vi "Estrai DB DW Contigui.vi"(10 "DB REAL LETTURE":T1(array[cluster])) -> (1 "DBW number":i32[](array[numeric]), 2 "DB offset":i32[](array[numeric]), 3 "DB":i16[](array[numeric]))   [LabVIEW 2019]
panel:
  out "x = y?":bool
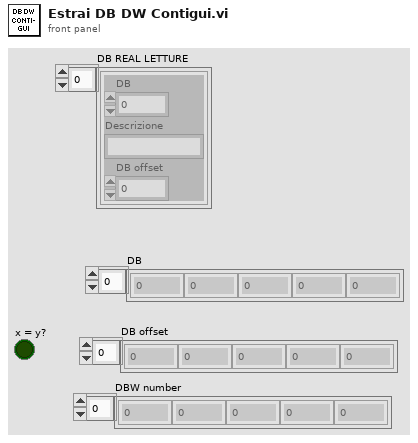
[diagram p1: front panel]
types:
  T1 = cluster{"DB":i16, "Descrizione":string, "DB offset":i16}[]
  T2 = cluster{"DB":i16, "Descrizione":string, "DB offset":i16}
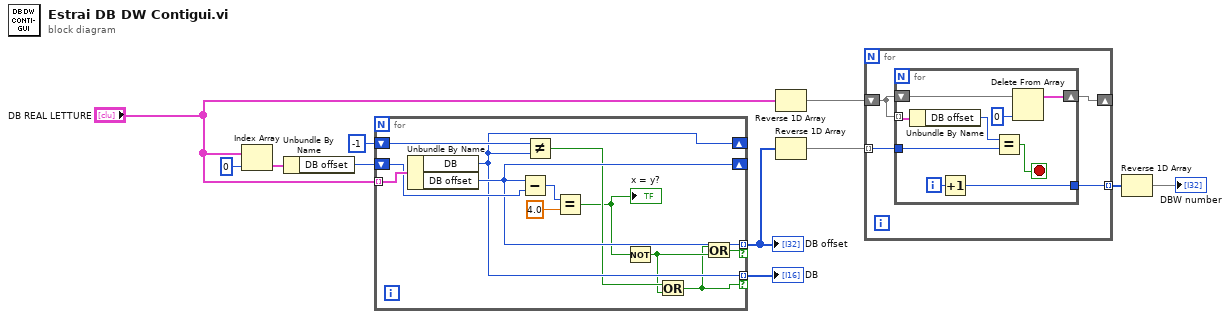
[diagram p0: block diagram]
diagram:
  n1 = Index Array(array="DB REAL LETTURE", index=0) -> (element=w10:T2)
  n2 = Unbundle By Name(w10) -> ("DB offset"=w9:i16)
  n3 = for {
    tunnel: "DB REAL LETTURE" -> [w23] mode=indexing
    shift-right: [w19] -> _
    shift-left: w9 -> [w22]
    tunnel: [w19] -> w8 mode=indexing if=w12
    tunnel: [w17] -> w3 mode=indexing if=w13
    shift-right: [w17] -> _
    shift-left: i16 -1 ("DB") -> [w18]
    n4 = Unbundle By Name(w23) -> ("DB"=w17:i16, "DB offset"=w19:i16)
    n5 = Subtract(x=w19, y=w22) -> (x-y=w21:i16)
    n6 = Not Equal?(x=w18, y=w17) -> (x != y?=w16:bool)
    n7 = Equal?(x=w21, y=4.0) -> (x = y?=w15:bool)
    "x = y?" <- w15
    n8 = Not(x=w15) -> (.not. x?=w14:bool)
    n9 = Or(x=w16, y=w14) -> (x .or. y?=w13:bool)
    n10 = Or(x=w13, y=w14) -> (x .or. y?=w12:bool)
  }
  "DB offset" <- w8
  "DB" <- w3
  n11 = Reverse 1D Array(array="DB REAL LETTURE") -> (reversed array=w6:T1)
  n12 = Reverse 1D Array(array=w8) -> (reversed array=w7:i16[])
  n13 = for {
    tunnel: w7 -> [w27] mode=indexing
    shift-right: [w25] -> _
    shift-left: w6 -> [w26]
    tunnel: [w24] -> w5 mode=indexing
    n14 = for {
      tunnel: w26 -> [w36] mode=indexing
      tunnel: w27 -> [w34]
      shift-right: [w30] -> w25
      shift-left: w26 -> [w32]
      tunnel: [w28] -> w24
      i -> [w29]
      stop <- w33 stop-if-true
      n15 = Unbundle By Name(w36) -> ("DB offset"=w35:i16)
      n16 = Increment(x=w29) -> (x+1=w28:i32)
      n17 = Equal?(x=w35, y=w34) -> (x = y?=w33:bool)
      n18 = Delete From Array(array=w32, index=0) -> (array with subset deleted=w30:T1)  [unwired: 1 in, 1 out]
    }
  }
  n19 = Reverse 1D Array(array=w5) -> (reversed array=→"DBW number":i32[])
